vi "Get Process Library Actions.vi"(8 "error in (no error)":errorcluster {"code" format="Error %.0f"}, 11 "VIDoc Printer In":refnum<class "VIDoc Printer.lvclass">) -> (0 "error out":errorcluster {"code" format="Error %.0f"}, 2 "Process Library Actions":T1[](array[typedef]), 3 "VIDoc Printer Out":refnum<class "VIDoc Printer.lvclass">)   [LabVIEW 2023, in "VIDoc Printer.lvlib" / "VIDoc Printer.lvclass"]
uses:
  VIDoc Printer.lvclass
  Controls/Process Library Enum.ctl
  VIDoc Printer.lvclass/VIDoc Printer.ctl
  Get Library Settings - Memory.vi
  Get Library Settings - By Folder.vi
  Get Library Settings - By Tree.vi
  Get Library Settings - By List.vi
  Get Library Settings - List Detail Level.vi
  Get Library Settings - Details.vi
  Get Library Settings - Detail Options - Description.vi
  Get Library Settings - Detail Options - Properties.vi
  Get Child Libraries.vi
  Get Library Settings - Detail Options - Friends.vi
  Get Library Settings - Methods Detail Level.vi
  Get Library Settings - Controls Detail Level.vi
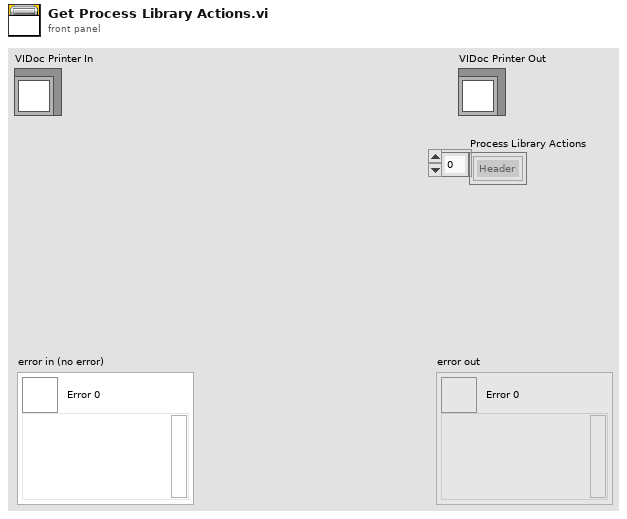
[diagram p1: front panel]
types:
  T1 = typedef "VIDoc Printer.lvlib/VIDoc Printer.lvclass/Process Library Enum.ctl" = enum16{"Header", "Memory", "By Folder", "By Tree", "By List", "Description", "Properties", "Child Libraries", "Friends", "Methods", "Controls"}
  T2 = typedef "VIDoc Printer.lvlib/Printer Settings.lvclass/Detail Level Enum.ctl" = enum16{"None", "Minimal", "Standard", "Full"}
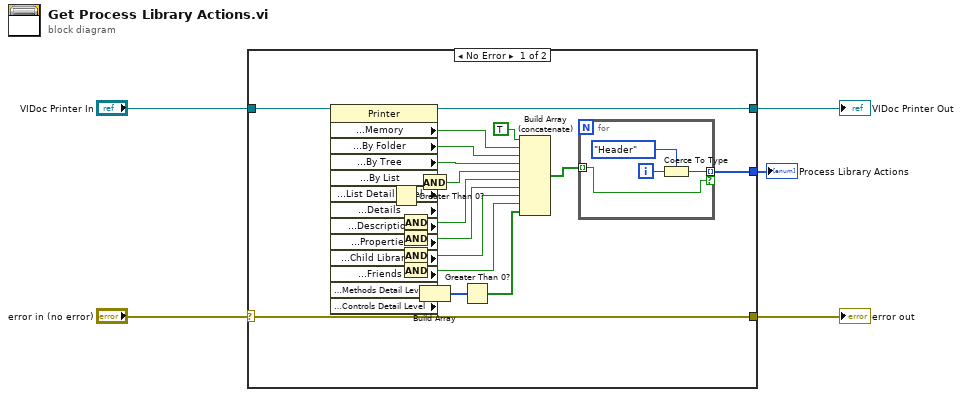
[diagram p0: block diagram]
diagram:
  n1 = case shown="No Error" "error in (no error)" {
    selector: "error in (no error)" -> [w31 w37]
    tunnel: [w31 w37] -> w4
    tunnel: [w20 w36] -> w2
    tunnel: "VIDoc Printer In" -> [w21 w36]
    tunnel: [w18 _] -> w1
    frame No Error {
      n2 = property class="Printer"(reference=w21) -> (reference out=w20:refnum<class "VIDoc Printer.lvclass">, "Properties:Settings:Libraries:Memory"=w25:bool, "Properties:Settings:Libraries:By Folder"=w24:bool, "Properties:Settings:Libraries:By Tree"=w23:bool, "Properties:Settings:Libraries:By List"=w22:bool, "Properties:Settings:Libraries:List Detail Level"=w17:T2, "Properties:Settings:Libraries:Details"=w8:bool, "Properties:Settings:Libraries:Description"=w14:bool, "Properties:Settings:Libraries:Properties"=w12:bool, "Properties:Settings:Libraries:Child Libraries"=w7:bool, "Properties:Settings:Libraries:Friends"=w11:bool, "Properties:Settings:Libraries:Methods Detail Level"=w29:T2, "Properties:Settings:Libraries:Controls Detail Level"=w28:T2)  [unwired: 1 in, 1 out]
      n3 = Greater Than 0?(x=w17) -> (x > 0?=w15:bool)
      n4 = And(x=w8, y=w14) -> (x .and. y?=w13:bool)
      n5 = And(x=w8, y=w12) -> (x .and. y?=w10:bool)
      n6 = And(x=w8, y=w7) -> (x .and. y?=w6:bool)
      n7 = And(x=w8, y=w11) -> (x .and. y?=w9:bool)
      n8 = And(x=w22, y=w15) -> (x .and. y?=w16:bool)
      n9 = Build Array(w29, w28) -> (w27:T2[])
      n10 = Greater Than 0?(x=w27) -> (x > 0?=w30:bool[])
      n11 = Build Array (concatenate)(TRUE ("element"), w25, w24, w23, w16, w13, w10, w6, w9, w30) -> (w19:bool[])
      n12 = for {
        tunnel: w19 -> [w32] mode=indexing
        tunnel: [w33] -> w18 mode=indexing if=w32
        i -> [w34]
        n13 = Coerce To Type(0:w34, 1:Process_Library_Enum."Header") -> (2:w33:T1)
      }
    }
    frame Error {
    }
  }
  "error out" <- w4
  "VIDoc Printer Out" <- w2
  "Process Library Actions" <- w1
